vi "Stop AWG.vi"(8 "error in (no error)":errorcluster, 10 "Pins":string[](array[string]), 11 "Semiconductor Module Context":T1) -> (0 "error out":errorcluster, 3 "Semiconductor Module Context Out":T1)   [LabVIEW 2013]
uses:
  <vilib>/NI_TestStand_SemiconductorModule/NI_TestStand_Semiconductor_Module.lvlibp/PinMap/General/SemiconductorModuleContext.ctl
  <vilib>/NI_TestStand_SemiconductorModule/NI_TestStand_Semiconductor_Module.lvlibp
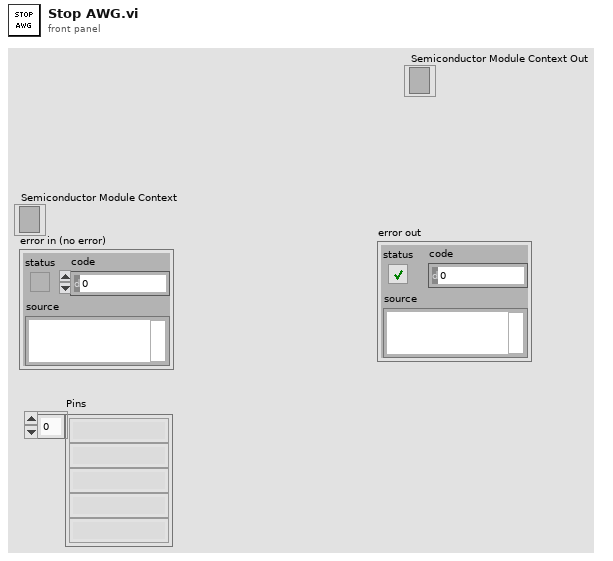
[diagram p1: front panel]
types:
  T1 = typedef "NI_TestStand_Semiconductor_Module.lvlibp/SemiconductorModuleContext.ctl" = refnum<k7>
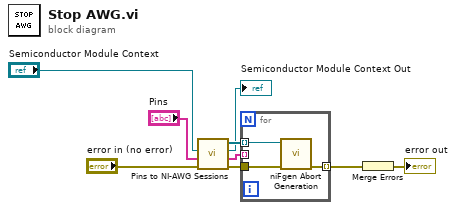
[diagram p0: block diagram]
diagram:
  n1 = call "Pins to NI-AWG Sessions.vi"("error in (no error)"="error in (no error)", "Pins"="Pins", "Semiconductor Module Context"="Semiconductor Module Context") -> ("error out"=w4:errorcluster, "Channel Lists"=w5:string[], "Semiconductor Module Context Out"=→"Semiconductor Module Context Out":T1, "Instrument Sessions"=w6:refnum<k15>[])  [unwired: 5 in]
  n2 = for {
    tunnel: w6 -> [w10] mode=indexing
    tunnel: w5 -> [_] mode=indexing
    tunnel: w4 -> [w12]
    tunnel: [w11] -> w3 mode=indexing
    n3 = call <instrlib>:"niFgen Abort Generation.vi"("error in (no error)"=w12, "Instrument Handle"=w10) -> ("error out"=w11:errorcluster)  [unwired: 8 in, 1 out]
  }
  n4 = Merge Errors(w3) -> (→"error out":errorcluster)
